vi "Write Experiment to TDMS Conversion Log.vi"(8 "error in (no error)":errorcluster, 10 "Additional Notes?":string, 11 "Conversion.lvclass":refnum<class "Conversion.lvclass">) -> (0 "error out":errorcluster, 2 "Log File Path":path, 3 "Conversion.lvclass out":refnum<class "Conversion.lvclass">)   [LabVIEW 2020, in "Conversion.lvclass"]
uses:
  Conversion.lvclass
  Conversion.lvclass/Conversion.ctl
  <userlib>/_OpenG.lib/array/array.llb/Remove Duplicates from 1D Array (Path)__ogtk.vi
  <userlib>/_OpenG.lib/file/file.llb/Strip Path - Arrays__ogtk.vi
panel:
  in  "OK":bool
  out "resulting string":string
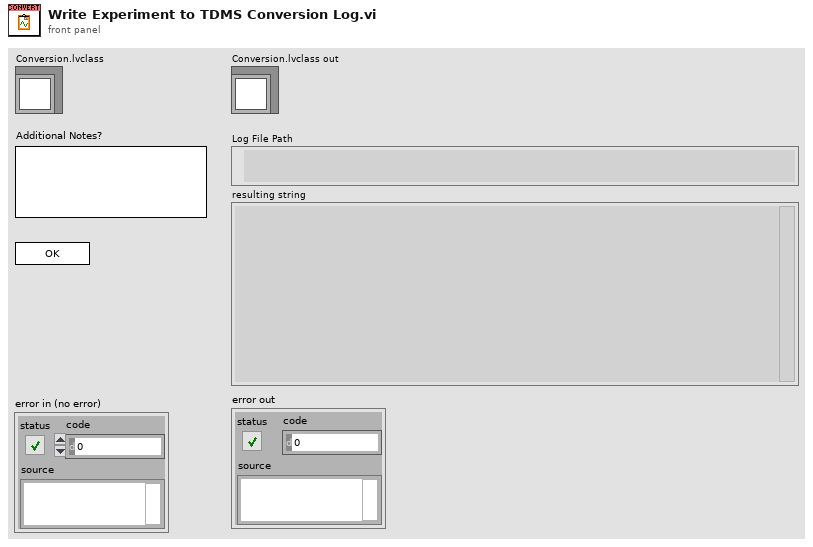
[diagram p1: front panel]
types:
  T1 = enum32{"Invalid", "Standard", "Closed", "Hidden", "Minimized", "Maximized"}
  T2 = enum32{"invalid app kind", "Development System", "Run Time System", "Student Edition", "Embedded LabVIEW", "Evaluation", "Custom"}
  T3 = cluster{"Core":cluster{"Current VI Reference":refnum<vi>, "Close Panel on Exit?":bool}, "Conversion.lvclass":refnum<class "Conversion.lvclass">, "Data.lvclass":refnum<class "Data.lvclass">, "Conversion Start time":timestamp, "Conversion End time":timestamp, "Archive End time":timestamp, "Original":path[], "Converted":path[], "Failed Conversions":path[], "Metadata":cluster{"Instrument":string, "Device":string, "Sample":string, "Experiment":string}, "Log":cluster{"Start Time":string, "Convert End Time":string, "Archive End Time":string, "string":string}}
  T4 = cluster{"Instrument":string, "Device":string, "Sample":string, "Experiment":string}
  T5 = cluster{"Start Time":string, "Convert End Time":string, "Archive End Time":string, "string":string}
  T6 = cluster{"Current VI Reference":refnum<vi>, "Close Panel on Exit?":bool}
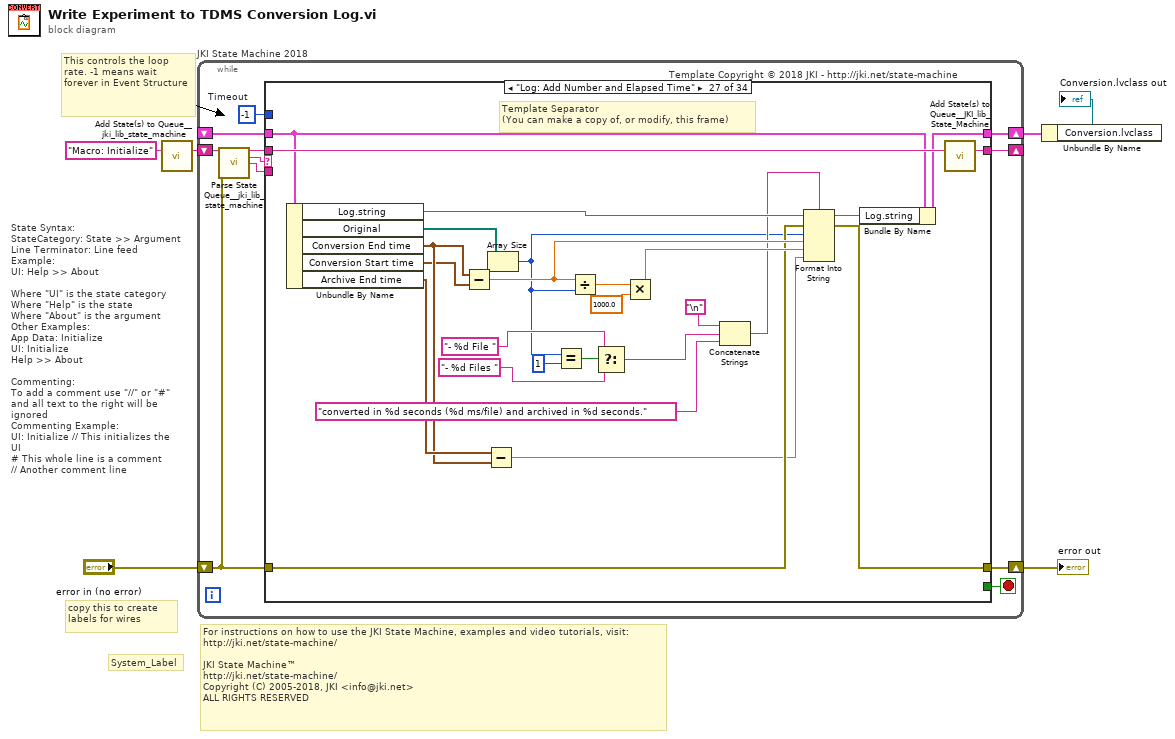
[diagram p0: block diagram]
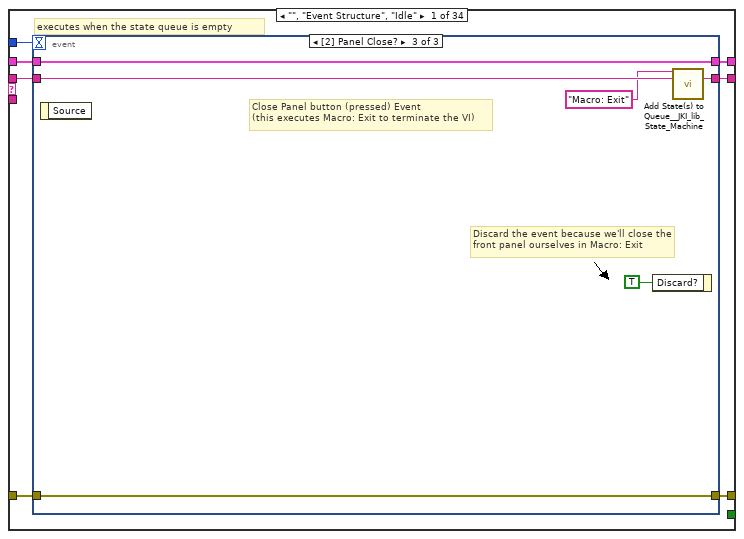
[diagram p2: hidden frame]
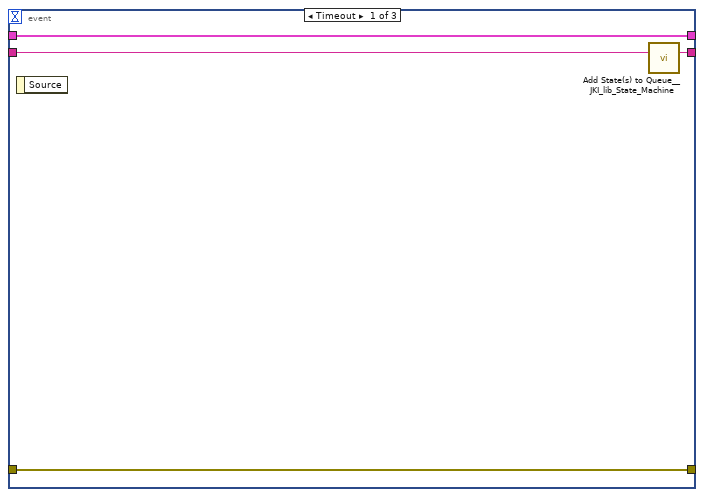
[diagram p3: hidden frame]
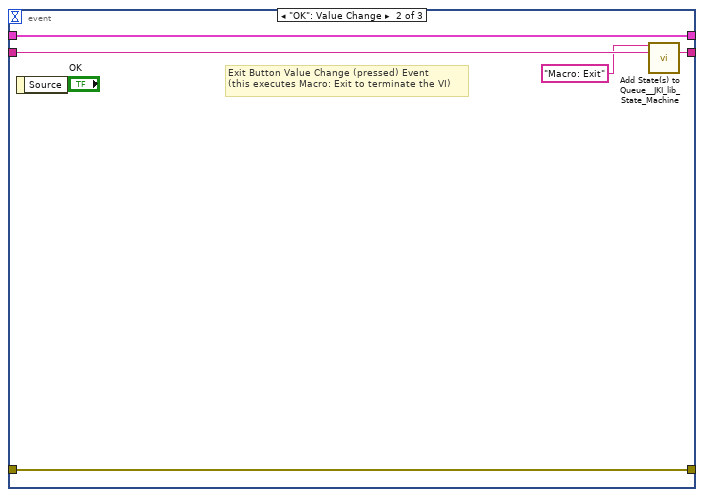
[diagram p4: hidden frame]
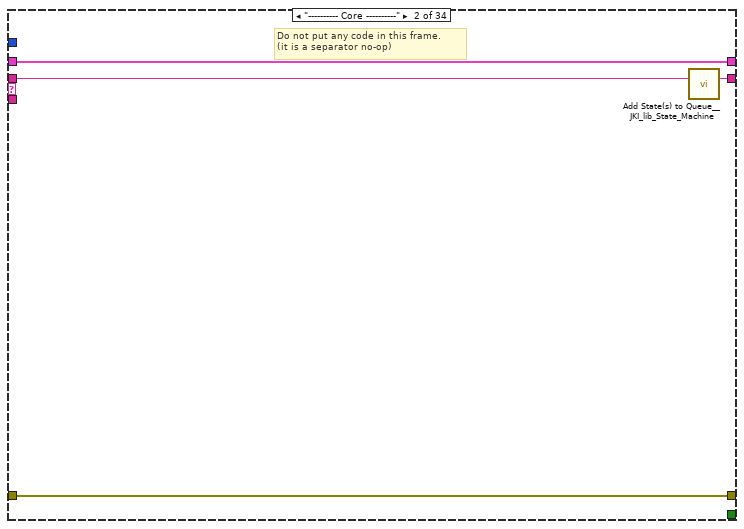
[diagram p5: hidden frame]
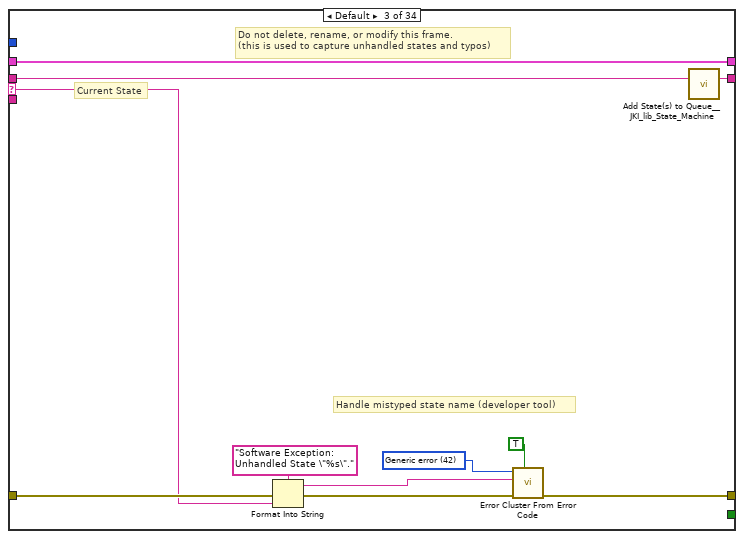
[diagram p6: hidden frame]
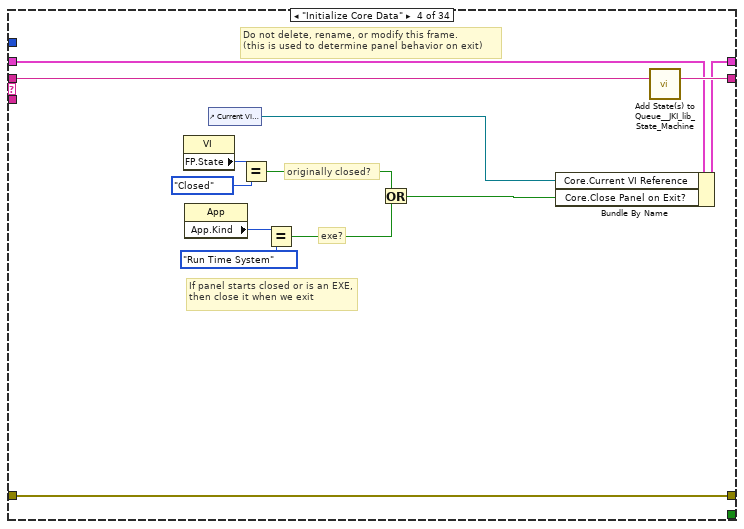
[diagram p7: hidden frame]
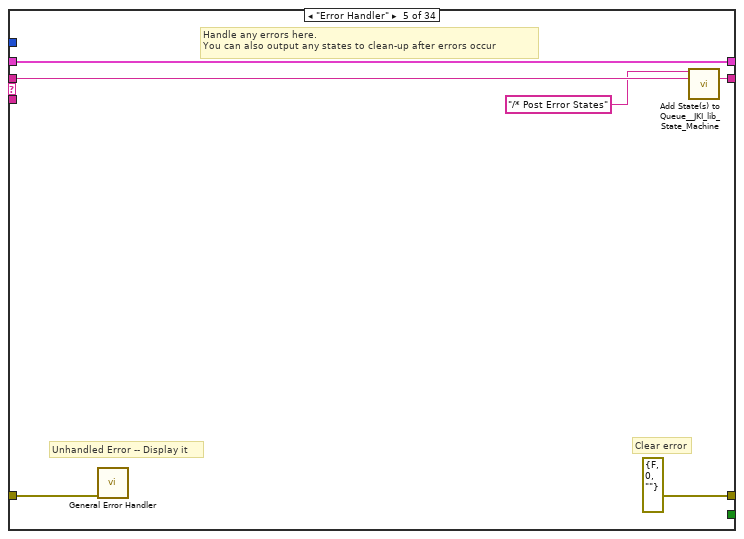
[diagram p8: hidden frame]
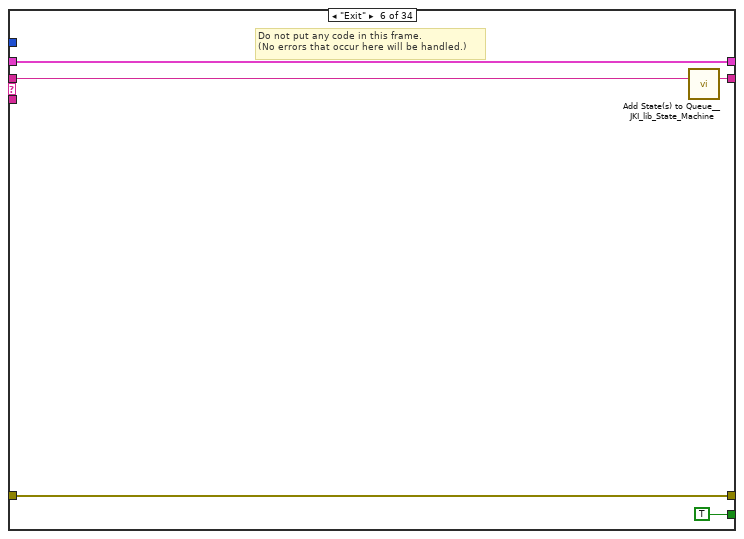
[diagram p9: hidden frame]
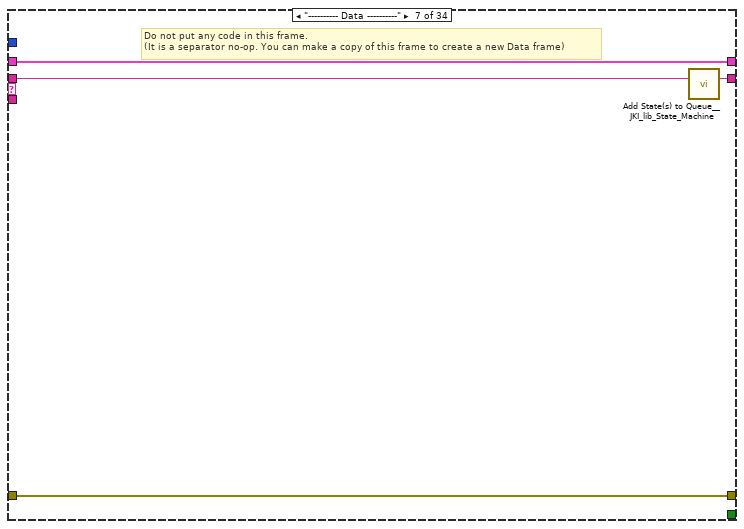
[diagram p10: hidden frame]
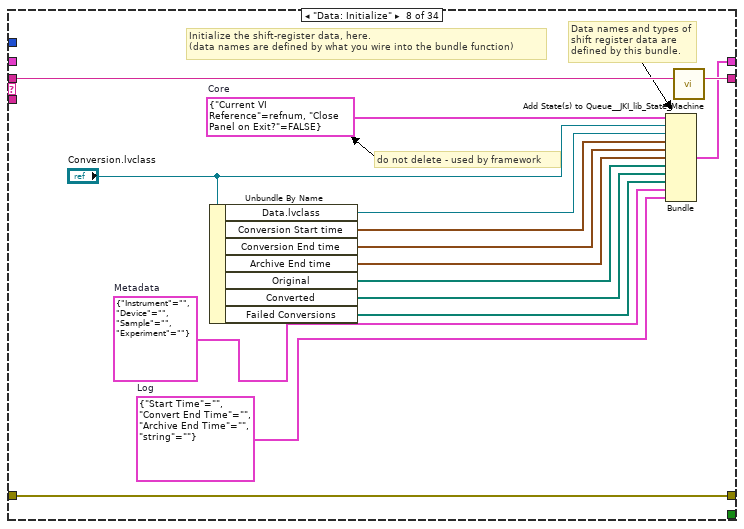
[diagram p11: hidden frame]
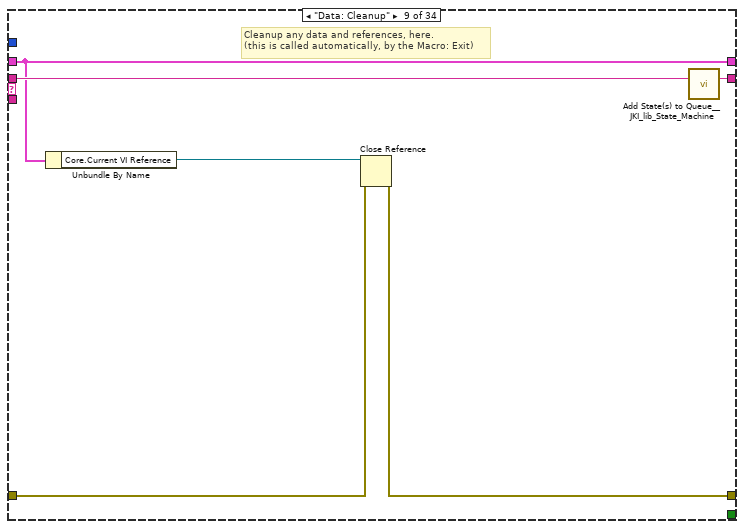
[diagram p12: hidden frame]
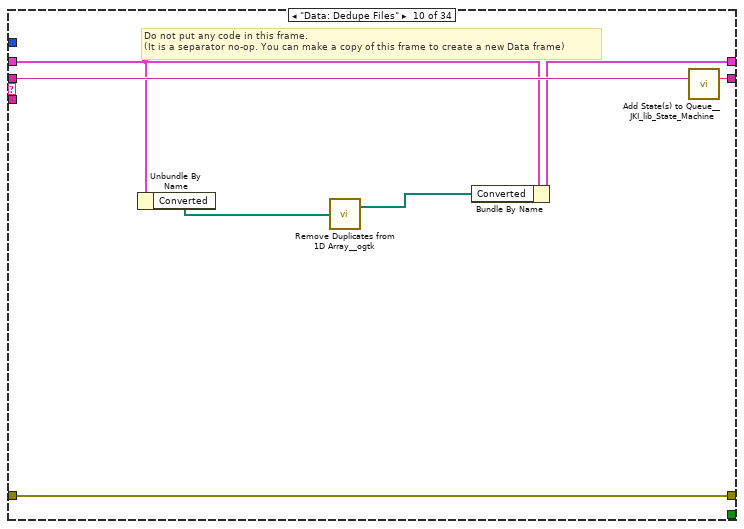
[diagram p13: hidden frame]
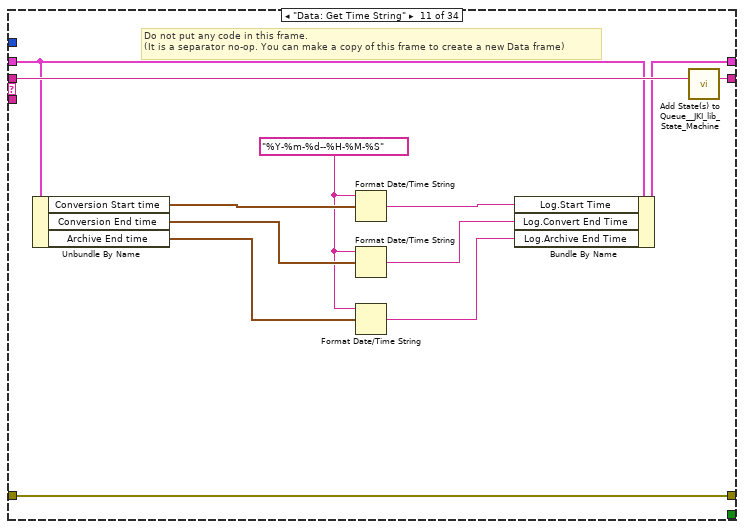
[diagram p14: hidden frame]
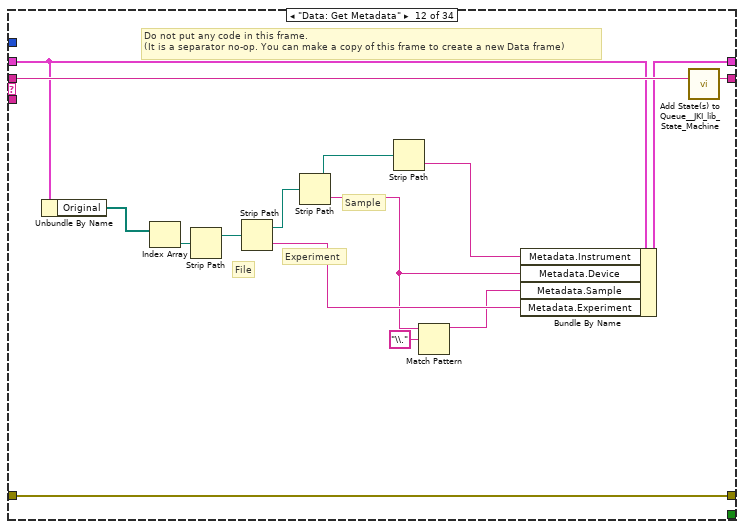
[diagram p15: hidden frame]
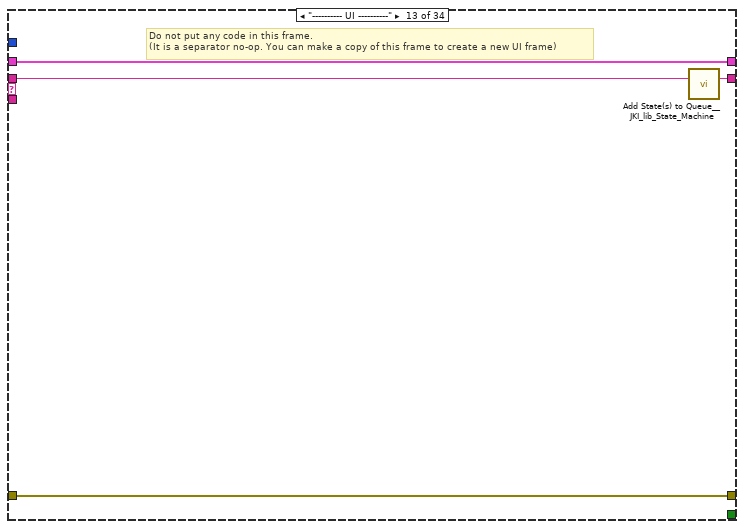
[diagram p16: hidden frame]
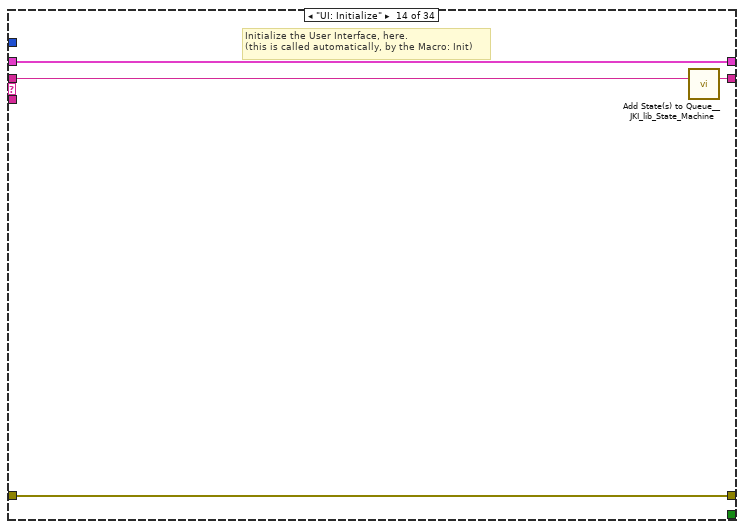
[diagram p17: hidden frame]
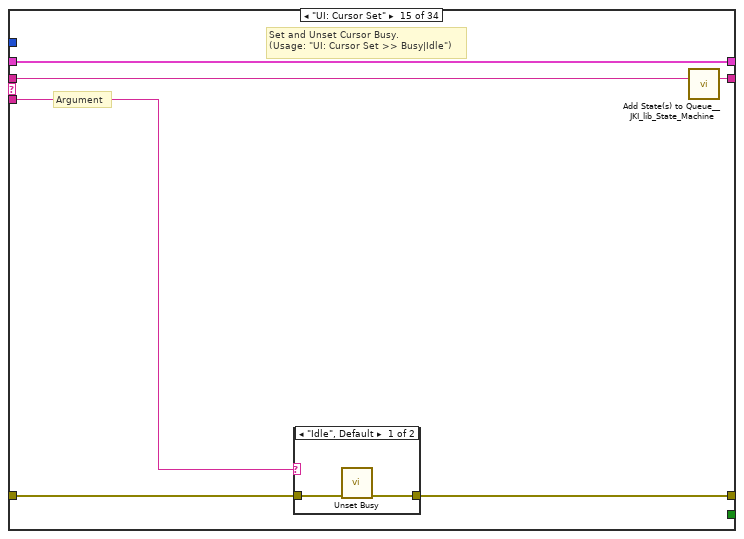
[diagram p18: hidden frame]
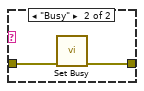
[diagram p19: hidden frame]
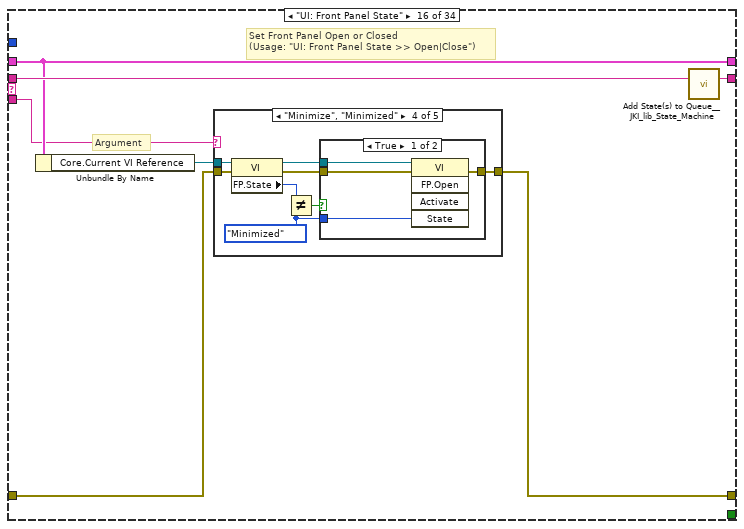
[diagram p20: hidden frame]
diagram:
  # "For instructions on how to use the JKI State Machine, examples and video tutorials, visit:\nhttp://jki.net/state-machine/\n\nJKI State Machine™\nhttp://jki.net/state-machine/\nCopyright (C) 2005-2018, JKI <info@jki.net>\nALL RIGHTS RESERVED"
  # "State Syntax:\nStateCategory: State >> Argument\nLine Terminator: Line feed\nExample:\nUI: Help >> About\n\nWhere \"UI\" is the state category\nWhere \"Help\" is the state\nWhere \"About\" is the argument\nOther Examples:\nApp Data: Initialize\nUI: Initialize\nHelp >> About\n\nCommenting:\nTo add a comment use \"//\" or \"#\" and all text to the right will be ignored\nCommenting Example:\nUI: Initialize // This initializes the UI\n# This whole line is a comment\n// Another comment line"
  # "copy this to create labels for wires"
  # "This controls the loop rate. -1 means wait forever in Event Structure"
  # "System_Label"
  n1 = call <vilib>:"Add State(s) to Queue__jki_lib_state_machine.vi"("State(s) in (\"\")"="Macro: Initialize") -> ("States Out"=w6:string)  [unwired: 14 in]
  n2 = while "JKI State Machine 2018" {
    shift-right: [w11] -> w2
    shift-left: _ -> [w10]
    shift-right: [w7] -> w4
    shift-left: "error in (no error)" -> [w8]
    shift-right: [w13] -> _
    shift-left: w6 -> [w14]
    stop <- w12 stop-if-true
    w9 = -1  # Timeout
    # "Template Copyright © 2018 JKI - http://jki.net/state-machine"
    n3 = call <vilib>:"Parse State Queue__jki_lib_state_machine.vi"("State Queue"=w14, "Error In (no error)"=w8) -> ("Remaining States"=w16:string, "Current State"=w17:string, "Arguments"=w15:string)  [unwired: 11 in]
    n4 = case shown="\"Log: Add Number and Elapsed Time\"" w17 {
      selector: w17 -> [_ _ w44 _ _ _ _ _ _ _ _ _ _ _ _ _ _ _ _ _ _ _ _ _ _ _ _ _ _ _ _ _ _ _]
      tunnel: w16 -> [w24 w43 w48 w67 w73 w78 w82 w97 w103 w110 w122 w137 w141 w145 w151 w162 w231 w236 w241 w251 w261 w265 w271 w281 w291 w301 w327 w339 w353 w388 w429 w447 w482 w508]
      tunnel: w15 -> [_ _ _ _ _ _ _ _ _ _ _ _ _ _ w146 w156 _ _ _ _ _ _ _ _ _ _ _ _ _ _ _ _ _ _]
      tunnel: w10 -> [w22 w40 w46 w60 w70 w76 w79 _ w98 w107 w119 w129 w138 w143 w149 w158 w228 w233 w238 w248 w259 w262 w268 w279 w289 w299 w325 w337 w351 w386 w427 w445 w480 w506]
      tunnel: w8 -> [w20 w41 w49 w64 w69 w75 w80 w94 w100 w108 w120 w135 w139 w142 w148 w160 w229 w234 w239 w249 w254 w263 w269 w273 w283 w293 w315 w332 w340 w381 w411 w441 w476 w497]
      tunnel: [w23 w42 w47 w66 w72 w77 w81 w96 w102 w109 w121 w136 w140 w144 w150 w161 w230 w235 w240 w250 w260 w264 w270 w280 w290 w300 w326 w338 w352 w387 w428 w446 w481 w507] -> w13
      tunnel: [_ _ _ _ _ TRUE _ _ _ _ _ _ _ _ _ _ _ _ _ _ _ _ _ _ _ _ _ _ _ _ _ _ _ _] -> w12
      tunnel: [w19 w40 w46 w65 w70 w76 w79 w95 w98 w105 w116 w128 w138 w143 w149 w158 w228 w233 w238 w248 w258 w262 w267 w278 w288 w298 w324 w336 w350 w385 w426 w444 w479 w506] -> w11
      tunnel: w9 -> [w18 _ _ _ _ _ _ _ _ _ _ _ _ _ _ _ _ _ _ _ _ _ _ _ _ _ _ _ _ _ _ _ _ _]
      tunnel: [w21 w41 w50 w64 errorcluster {"status"=FALSE, "code"=0, "source"=""} ("error out") w75 w80 w94 w99 w108 w120 w135 w139 w142 w147 w159 w229 w234 w239 w249 w253 w263 w269 w274 w282 w292 w316 w331 w346 w383 w422 w436 w475 w502] -> w7
      frame "", "Event Structure", "Idle" {
        # "executes when the state queue is empty"
        n5 = event shown="[2] Panel Close?" {
          selector: _ -> [_ _ _]
          dyn-events: _ -> [_ _ _]
          timeout: w18 -> [_ _ _]
          tunnel: w24 -> [w28 w33 w39]
          tunnel: [w27 w32 w38] -> w23
          tunnel: w22 -> [w25 w30 w36]
          tunnel: [w26 w31 w37] -> w21
          tunnel: w20 -> [w26 w31 w37]
          tunnel: [w25 w30 w36] -> w19
          event Timeout {
            n6 = event-data() -> ()  [unwired: 1 in, 1 out]
            n7 = call <vilib>:"Add State(s) to Queue__JKI_lib_State_Machine.vi"("State(s) in (\"\")"=w28) -> ("States Out"=w27:string)  [unwired: 14 in]
          }
          event "OK": Value Change {
            # "Exit Button Value Change (pressed) Event\n(this executes Macro: Exit to terminate the VI)"
            n8 = event-data() -> ()  [unwired: 1 in, 1 out]
            n9 = call <vilib>:"Add State(s) to Queue__JKI_lib_State_Machine.vi"("State(s) in Front (\"\")"="Macro: Exit", "State(s) in (\"\")"=w33) -> ("States Out"=w32:string)  [unwired: 13 in]
          }
          event Panel Close? {
            # "Discard the event because we'll close the front panel ourselves in Macro: Exit"
            # "Close Panel button (pressed) Event\n(this executes Macro: Exit to terminate the VI)"
            n10 = event-data() -> ()  [unwired: 1 in, 1 out]
            n11 = event-data("Discard?"=TRUE) -> ()  [unwired: 1 in, 1 out]
            n12 = call <vilib>:"Add State(s) to Queue__JKI_lib_State_Machine.vi"("State(s) in Front (\"\")"="Macro: Exit", "State(s) in (\"\")"=w39) -> ("States Out"=w38:string)  [unwired: 13 in]
          }
        }
      }
      frame "---------- Core ----------" {
        # "Do not put any code in this frame.\n(it is a separator no-op)"
        n13 = call <vilib>:"Add State(s) to Queue__JKI_lib_State_Machine.vi"("State(s) in (\"\")"=w43) -> ("States Out"=w42:string)  [unwired: 14 in]
      }
      frame Default {
        w53 = 42 items=["No error", "Argument error", "Memory is full", "Out of zone", "End of file", "File already open", "Generic file I/O error", "File not found", "File permission error", "Disk is full", "Duplicate path", "Too many files open", "System feature not enabled", "Resource file not found", "Cannot add resource", "Resource not found", "Image not found", "Image memory error", "Pen does not exist", "Config type invalid", "Config token not found", "Config parse error", "Config memory error", "Bad external code format", "Bad external code offset", "External code not present", "Null window", "Destroy window error", "Null menu", "Print aborted", "Bad print record", "Print driver error", "Windows error during printing", "Memory error during printing", "Print dialog error", "Generic print error", "Invalid device refnum", "Device not found", "Device parameter error", "Device unit error", "Cannot open device", "Device call aborted", "Generic error", "Cancelled by user", "Object ID too low", "Object ID too high", "Object not in heap", "Unknown heap", "Unknown object (invalid DefProc)", "Unknown object (DefProc not in table)", "Message out of range", "Invalid (null) method", "Unknown message", "Manager call not supported", "Bad address", "Network operation in progress", "Network operation timed out", "Connection is busy", "Network attribute not supported", "Network error", "Address in use", "System out of memory", "Connection aborted", "Connection refused", "Not connected", "Already connected", "Connection closed", "Initialization error (interapplication manager)", "Bad occurrence", "Wait on unbound occurrence handler", "Occurrence queue overflow", "Datalog type conflict", "Unused", "Unrecognized type (interapplication manager)", "Memory corrupt", "Failed to make temporary DLL", "Old CIN version", "Drag socket not found", "Failed to load drop-object", "Failed to register OLE object", "Failed to release OLE object", "Format specifier type mismatch", "Unknown format specifier", "Too few format specifiers", "Too many format specifiers", "Scan failed", "Newer CIN version", "Error converting to variant", "Runtime menu error", "Password tampered", "Variant attribute not found", "Incompatible variant data type", "Event data is not available", "Event Store is not present", "Occurrence is not found", "Event Queue is not created", "Event info is not available", "Refnum passed is NULL", "Error retrieving Class GUID", "Error retrieving CoClass GUID", "Error retrieving TypeLib GUID.", "Bad built application magic bytes.", "Specific driver is different from the specific driver associated with the Logical Name.", "There is no session opened to the class driver.", "Max Error", "MAX - Error with config objects", "MAX - Error loading configuration", "MAX - Group not supported"]
        # "Current State"
        # "Do not delete, rename, or modify this frame.\n(this is used to capture unhandled states and typos)"
        # "Handle mistyped state name (developer tool)"
        n14 = Format Into String(format string="Software Exception: Unhandled State \"%s\"." ("message"), error in=w49, w44) -> (resulting string=w52:string, error out=w51:errorcluster)  [unwired: 1 in]
        n15 = call <vilib>:"Error Cluster From Error Code.vi"("show call chain? (False)"=TRUE, "error in (no error)"=w51, "error message (\"\")"=w52, "error code (0)"=w53) -> ("error out"=w50:errorcluster)  [unwired: 5 in]
        n16 = call <vilib>:"Add State(s) to Queue__JKI_lib_State_Machine.vi"("State(s) in (\"\")"=w48) -> ("States Out"=w47:string)  [unwired: 14 in]
      }
      frame "Initialize Core Data" {
        # "Do not delete, rename, or modify this frame.\n(this is used to determine panel behavior on exit)"
        # "originally closed?"
        # "exe?"
        # "If panel starts closed or is an EXE, then close it when we exit"
        n17 = property class="VI"() -> ("FP.State"=w57:T1)  [unwired: 2 in, 2 out]
        n18 = property class="App"() -> ("App.Kind"=w63:T2)  [unwired: 2 in, 2 out]
        n19 = control-ref of="Current VI Reference"() -> (w58:refnum<vi>)
        n20 = Equal?(x=w57, y=T1."Closed" ("Front Panel Window:State")) -> (x = y?=w55:bool)
        n21 = Equal?(x=w63, y=T2."Run Time System" ("Application:Kind")) -> (x = y?=w61:bool)
        n22 = Or(x=w55, y=w61) -> (x .or. y?=w59:bool)
        n23 = Bundle By Name(cluster=w60, "Core.Current VI Reference"=w58, "Core.Close Panel on Exit?"=w59) -> (w65:T3)
        n24 = call <vilib>:"Add State(s) to Queue__JKI_lib_State_Machine.vi"("State(s) in (\"\")"=w67) -> ("States Out"=w66:string)  [unwired: 14 in]
      }
      frame "Error Handler" {
        # "Unhandled Error -- Display it"
        # "Handle any errors here.\nYou can also output any states to clean-up after errors occur"
        # "Clear error"
        n25 = call <vilib>:"General Error Handler.vi"("error in (no error)"=w69) -> ()  [unwired: 10 in, 5 out]
        n26 = call <vilib>:"Add State(s) to Queue__JKI_lib_State_Machine.vi"("State(s) in Front (\"\")"="/* Post Error States", "State(s) in (\"\")"=w73) -> ("States Out"=w72:string)  [unwired: 13 in]
      }
      frame "Exit" {
        # "Do not put any code in this frame.\n(No errors that occur here will be handled.)"
        n27 = call <vilib>:"Add State(s) to Queue__JKI_lib_State_Machine.vi"("State(s) in (\"\")"=w78) -> ("States Out"=w77:string)  [unwired: 14 in]
      }
      frame "---------- Data ----------" {
        # "Do not put any code in this frame.\n(It is a separator no-op. You can make a copy of this frame to create a new Data frame)"
        n28 = call <vilib>:"Add State(s) to Queue__JKI_lib_State_Machine.vi"("State(s) in (\"\")"=w82) -> ("States Out"=w81:string)  [unwired: 14 in]
      }
      frame "Data: Initialize" {
        w84 = T4 {"Instrument"="", "Device"="", "Sample"="", "Experiment"=""}  # Metadata
        w85 = T5 {"Start Time"="", "Convert End Time"="", "Archive End Time"="", "string"=""}  # Log
        w93 = T6 {"Current VI Reference"=refnum, "Close Panel on Exit?"=FALSE}  # Core
        # "do not delete - used by framework"
        # "Data names and types of shift register data are defined by this bundle."
        # "Initialize the shift-register data, here.\n(data names are defined by what you wire into the bundle function)"
        n29 = Unbundle By Name("Conversion.lvclass") -> ("Data.lvclass"=w92:refnum<class "Data.lvclass">, "Conversion Start time"=w91:timestamp, "Conversion End time"=w90:timestamp, "Archive End time"=w86:timestamp, "Original"=w88:path[], "Converted"=w87:path[], "Failed Conversions"=w89:path[])
        n30 = Bundle("Core"=w93, "Conversion.lvclass"="Conversion.lvclass", "Data.lvclass"=w92, "Conversion Start time"=w91, "Conversion End time"=w90, "Archive End time"=w86, "Original"=w88, "Converted"=w87, "Failed Conversions"=w89, "Metadata"=w84, "Log"=w85) -> (w95:T3)  [unwired: 1 in]
        n31 = call <vilib>:"Add State(s) to Queue__JKI_lib_State_Machine.vi"("State(s) in (\"\")"=w97) -> ("States Out"=w96:string)  [unwired: 14 in]
      }
      frame "Data: Cleanup" {
        # "Cleanup any data and references, here.\n(this is called automatically, by the Macro: Exit)"
        n32 = Unbundle By Name(w98) -> ("Core.Current VI Reference"=w101:refnum<vi>)
        n33 = Close Reference(reference=w101, error in (no error)=w100) -> (error out=w99:errorcluster)
        n34 = call <vilib>:"Add State(s) to Queue__JKI_lib_State_Machine.vi"("State(s) in (\"\")"=w103) -> ("States Out"=w102:string)  [unwired: 14 in]
      }
      frame "Data: Dedupe Files" {
        # "Do not put any code in this frame.\n(It is a separator no-op. You can make a copy of this frame to create a new Data frame)"
        n35 = Unbundle By Name(w107) -> ("Converted"=w106:path[])
        n36 = call-poly <userlib>:"Remove Duplicates from 1D Array__ogtk.vi"("Input Array"=w106) -> ("Output Array"=w104:path[])  [unwired: 1 out]
        n37 = Bundle By Name(cluster=w107, "Converted"=w104) -> (w105:T3)
        n38 = call <vilib>:"Add State(s) to Queue__JKI_lib_State_Machine.vi"("State(s) in (\"\")"=w110) -> ("States Out"=w109:string)  [unwired: 14 in]
      }
      frame "Data: Get Time String" {
        w112 = "%Y-%m-%d--%H-%M-%S" ("time format string (%c)")
        # "Do not put any code in this frame.\n(It is a separator no-op. You can make a copy of this frame to create a new Data frame)"
        n39 = Unbundle By Name(w119) -> ("Conversion Start time"=w118:timestamp, "Conversion End time"=w117:timestamp, "Archive End time"=w113:timestamp)
        n40 = Format Date/Time String(time format string (%c)=w112, seconds (now)=w118) -> (date/time string=w115:string)  [unwired: 1 in]
        n41 = Format Date/Time String(time format string (%c)=w112, seconds (now)=w117) -> (date/time string=w114:string)  [unwired: 1 in]
        n42 = Format Date/Time String(time format string (%c)=w112, seconds (now)=w113) -> (date/time string=w111:string)  [unwired: 1 in]
        n43 = Bundle By Name(cluster=w119, "Log.Start Time"=w115, "Log.Convert End Time"=w114, "Log.Archive End Time"=w111) -> (w116:T3)
        n44 = call <vilib>:"Add State(s) to Queue__JKI_lib_State_Machine.vi"("State(s) in (\"\")"=w122) -> ("States Out"=w121:string)  [unwired: 14 in]
      }
      frame "Data: Get Metadata" {
        # "Sample"
        # "Experiment"
        # "File"
        # "Do not put any code in this frame.\n(It is a separator no-op. You can make a copy of this frame to create a new Data frame)"
        n45 = Unbundle By Name(w129) -> ("Original"=w130:path[])
        n46 = Index Array(array=w130) -> (element=w133:path)  [unwired: 1 in]
        n47 = Strip Path(path=w133) -> (stripped path=w132:path)  [unwired: 1 out]
        n48 = Strip Path(path=w132) -> (stripped path=w134:path, name=w126:string)
        n49 = Strip Path(path=w134) -> (stripped path=w131:path, name=w125:string)
        n50 = Strip Path(path=w131) -> (name=w127:string)  [unwired: 1 out]
        n51 = Match Pattern(string=w125, regular expression="\\.") -> (before substring=w123:string)  [unwired: 1 in, 3 out]
        n52 = Bundle By Name(cluster=w129, "Metadata.Instrument"=w127, "Metadata.Device"=w125, "Metadata.Sample"=w123, "Metadata.Experiment"=w126) -> (w128:T3)
        n53 = call <vilib>:"Add State(s) to Queue__JKI_lib_State_Machine.vi"("State(s) in (\"\")"=w137) -> ("States Out"=w136:string)  [unwired: 14 in]
      }
      frame "---------- UI ----------" {
        # "Do not put any code in this frame.\n(It is a separator no-op. You can make a copy of this frame to create a new UI frame)"
        n54 = call <vilib>:"Add State(s) to Queue__JKI_lib_State_Machine.vi"("State(s) in (\"\")"=w141) -> ("States Out"=w140:string)  [unwired: 14 in]
      }
      frame "UI: Initialize" {
        # "Initialize the User Interface, here.\n(this is called automatically, by the Macro: Init)"
        n55 = call <vilib>:"Add State(s) to Queue__JKI_lib_State_Machine.vi"("State(s) in (\"\")"=w145) -> ("States Out"=w144:string)  [unwired: 14 in]
      }
      frame "UI: Cursor Set" {
        # "Argument"
        # "Set and Unset Cursor Busy.\n(Usage: \"UI: Cursor Set >> Busy|Idle\")"
        n56 = case shown="\"Idle\", Default" w146 {
          tunnel: w148 -> [w153 w155]
          tunnel: [w152 w154] -> w147
          frame "Idle", Default {
            n57 = call <vilib>:"Unset Busy.vi"("error in (no error)"=w153) -> ("error out"=w152:errorcluster)  [unwired: 10 in]
          }
          frame "Busy" {
            n58 = call <vilib>:"Set Busy.vi"("error in (no error)"=w155) -> ("error out"=w154:errorcluster)  [unwired: 9 in, 1 out]
          }
        }
        n59 = call <vilib>:"Add State(s) to Queue__JKI_lib_State_Machine.vi"("State(s) in (\"\")"=w151) -> ("States Out"=w150:string)  [unwired: 14 in]
      }
      frame "UI: Front Panel State" {
        # "Argument"
        # "Set Front Panel Open or Closed\n(Usage: \"UI: Front Panel State >> Open|Close\")"
        n60 = Unbundle By Name(w158) -> ("Core.Current VI Reference"=w157:refnum<vi>)
        n61 = case shown="\"Minimize\", \"Minimized\"" w156 {
          tunnel: w160 -> [w168 w183 w194 w207 w220]
          tunnel: [w170 w184 w196 w209 w222] -> w159
          tunnel: w157 -> [w169 w181 w195 w208 w221]
          frame "Open", "Standard", Default {
            w163 = T1."Standard" ("State")
            n62 = property class="VI"(reference=w169, error in=w168) -> (reference out=w166:refnum<vi>, error out=w167:errorcluster, "FP.State"=w165:T1)
            n63 = Not Equal?(x=w165, y=w163) -> (x != y?=w164:bool)
            n64 = case shown="True" w164 {
              tunnel: [w174 w176] -> w170
              tunnel: w167 -> [w173 w176]
              tunnel: w166 -> [w172 _]
              tunnel: w163 -> [w171 _]
              frame True {
                n65 = invoke class="VI" method="FP.Open"(reference=w172, error in=w173, "Activate"=TRUE, "State"=w171) -> (error out=w174:errorcluster)  [unwired: 1 in, 4 out]
              }
              frame False {
              }
            }
          }
          frame "Close", "Closed" {
            n66 = property class="VI"(reference=w181, error in=w183) -> (reference out=w180:refnum<vi>, error out=w182:errorcluster, "FP.State"=w178:T1)
            n67 = Not Equal?(x=w178, y=T1."Closed" ("Front Panel Window:State")) -> (x != y?=w177:bool)
            n68 = case shown="True" w177 {
              tunnel: [w185 w188] -> w184
              tunnel: w182 -> [w185 w187]
              tunnel: w180 -> [_ w186]
              frame False {
              }
              frame True {
                n69 = invoke class="VI" method="FP.Close"(reference=w186, error in=w187) -> (error out=w188:errorcluster)  [unwired: 1 in, 2 out]
              }
            }
          }
          frame "Hidden", "Hide" {
            w189 = T1."Hidden" ("State")
            n70 = property class="VI"(reference=w195, error in=w194) -> (reference out=w192:refnum<vi>, error out=w193:errorcluster, "FP.State"=w191:T1)
            n71 = Not Equal?(x=w191, y=w189) -> (x != y?=w190:bool)
            n72 = case shown="True" w190 {
              tunnel: [w200 w201] -> w196
              tunnel: w193 -> [w199 w201]
              tunnel: w192 -> [w198 _]
              tunnel: w189 -> [w197 _]
              frame True {
                n73 = invoke class="VI" method="FP.Open"(reference=w198, error in=w199, "State"=w197) -> (error out=w200:errorcluster)  [unwired: 2 in, 4 out]
              }
              frame False {
              }
            }
          }
          frame "Minimize", "Minimized" {
            w202 = T1."Minimized" ("State")
            n74 = property class="VI"(reference=w208, error in=w207) -> (reference out=w205:refnum<vi>, error out=w206:errorcluster, "FP.State"=w204:T1)
            n75 = Not Equal?(x=w204, y=w202) -> (x != y?=w203:bool)
            n76 = case shown="True" w203 {
              tunnel: [w213 w214] -> w209
              tunnel: w206 -> [w212 w214]
              tunnel: w205 -> [w211 _]
              tunnel: w202 -> [w210 _]
              frame True {
                n77 = invoke class="VI" method="FP.Open"(reference=w211, error in=w212, "State"=w210) -> (error out=w213:errorcluster)  [unwired: 2 in, 4 out]
              }
              frame False {
              }
            }
          }
          frame "Maximize", "Maximized" {
            w215 = T1."Maximized" ("State")
            n78 = property class="VI"(reference=w221, error in=w220) -> (reference out=w218:refnum<vi>, error out=w219:errorcluster, "FP.State"=w217:T1)
            n79 = Not Equal?(x=w217, y=w215) -> (x != y?=w216:bool)
            n80 = case shown="True" w216 {
              tunnel: [w226 w227] -> w222
              tunnel: w219 -> [w225 w227]
              tunnel: w218 -> [w224 _]
              tunnel: w215 -> [w223 _]
              frame True {
                n81 = invoke class="VI" method="FP.Open"(reference=w224, error in=w225, "State"=w223) -> (error out=w226:errorcluster)  [unwired: 2 in, 4 out]
              }
              frame False {
              }
            }
          }
        }
        n82 = call <vilib>:"Add State(s) to Queue__JKI_lib_State_Machine.vi"("State(s) in (\"\")"=w162) -> ("States Out"=w161:string)  [unwired: 14 in]
      }
      frame "---------- Macro ----------" {
        # "Do not put any code in this frame.\n(It is a separator no-op. You can make a copy of this frame to create a new Macro frame)"
        n83 = call <vilib>:"Add State(s) to Queue__JKI_lib_State_Machine.vi"("State(s) in (\"\")"=w231) -> ("States Out"=w230:string)  [unwired: 14 in]
      }
      frame "Macro: Initialize" {
        w232 = "Data: Initialize\nInitialize Core Data\nUI: Initialize\nUI: Front Panel State >> Open\nMacro: Log\nMacro: Exit"  # Data: Initialize Initialize Core Data UI: Initialize UI: Front Panel State >> Open Macro: Log Macro: Exit
        # "Initialization Macro\n(This is called once, when the VI starts)"
        n84 = call <vilib>:"Add State(s) to Queue__JKI_lib_State_Machine.vi"("State(s) in Front (\"\")"=w232, "State(s) in (\"\")"=w236) -> ("States Out"=w235:string)  [unwired: 13 in]
      }
      frame "Macro: Log" {
        # "Initialization Macro\n(This is called once, when the VI starts)"
        n85 = call <vilib>:"Add State(s) to Queue__JKI_lib_State_Machine.vi"("State(s) in Front (\"\")"="Log: Temp\nData: Dedupe Files\nData: Get Time String\nData: Get Metadata\nLog: Initialize\nLog: Add Start Time\nLog: Add Convert End Time\nLog: Add Archive End Time\nLog: Add Number and Elapsed Time\nLog: Add Original Folder Name\nLog: Add Converted Folder Name\nLog: Add Number of Files\nLog: Add File Sizes\nLog: Add Notes\nLog: Add Files\nLog: Write File", "State(s) in (\"\")"=w241) -> ("States Out"=w240:string)  [unwired: 13 in]
      }
      frame "Macro: Exit" {
        # "Exit Macro\n(This is called once, when the VI exits)"
        n86 = Unbundle By Name(w248) -> ("Core.Close Panel on Exit?"=w247:bool)
        n87 = Select(t="UI: Front Panel State >> Close", s=w247, f="") -> (s? t:f=w244:string)
        n88 = call <vilib>:"Add State(s) to Queue__JKI_lib_State_Machine.vi"("State(s) in (\"\")"=w244, "State(s) at Back (\"\")"="Data: Cleanup\nExit") -> ("States Out"=w242:string)  [unwired: 13 in]
        n89 = call <vilib>:"Add State(s) to Queue__JKI_lib_State_Machine.vi"("State(s) in Front (\"\")"=w242, "State(s) in (\"\")"=w251) -> ("States Out"=w250:string)  [unwired: 13 in]
      }
      frame "---------- Log ----------" {
        # "Template Separator\n(You can make a copy of, or modify, this frame)"
        n90 = Unbundle By Name(w259) -> ("Log.string"=w256:string)
        n91 = Format Into String(format string="\n%s", initial string=w256, error in=w254, "" ("input 1")) -> (resulting string=w255:string, error out=w253:errorcluster)
        n92 = Bundle By Name(cluster=w259, "Log.string"=w255) -> (w258:T3)
        n93 = call <vilib>:"Add State(s) to Queue__JKI_lib_State_Machine.vi"("State(s) in (\"\")"=w261) -> ("States Out"=w260:string)  [unwired: 14 in]
      }
      frame "Log: Temp" {
        # "Your code here.\n(You can make a copy of, or modify, this frame)"
        n94 = call <vilib>:"Add State(s) to Queue__JKI_lib_State_Machine.vi"("State(s) in (\"\")"=w265) -> ("States Out"=w264:string)  [unwired: 14 in]
      }
      frame "Log: Initialize" {
        w266 = "Data File Conversion Summary"  # new
        # "Template Separator\n(You can make a copy of, or modify, this frame)"
        n95 = Bundle By Name(cluster=w268, "Log.string"=w266) -> (w267:T3)
        n96 = call <vilib>:"Add State(s) to Queue__JKI_lib_State_Machine.vi"("State(s) in (\"\")"=w271) -> ("States Out"=w270:string)  [unwired: 14 in]
      }
      frame "Log: Add Start Time" {
        # "Template Separator\n(You can make a copy of, or modify, this frame)"
        n97 = Unbundle By Name(w279) -> ("Log.string"=w276:string, "Log.Start Time"=w272:string)
        n98 = Format Into String(format string="\n- Start Time: %s", initial string=w276, error in=w273, w272) -> (resulting string=w275:string, error out=w274:errorcluster)
        n99 = Bundle By Name(cluster=w279, "Log.string"=w275) -> (w278:T3)
        n100 = call <vilib>:"Add State(s) to Queue__JKI_lib_State_Machine.vi"("State(s) in (\"\")"=w281) -> ("States Out"=w280:string)  [unwired: 14 in]
      }
      frame "Log: Add Convert End Time" {
        # "Template Separator\n(You can make a copy of, or modify, this frame)"
        n101 = Unbundle By Name(w289) -> ("Log.string"=w286:string, "Log.Convert End Time"=w285:string)
        n102 = Format Into String(format string="\n- End Time: %s", initial string=w286, error in=w283, w285) -> (resulting string=w284:string, error out=w282:errorcluster)
        n103 = Bundle By Name(cluster=w289, "Log.string"=w284) -> (w288:T3)
        n104 = call <vilib>:"Add State(s) to Queue__JKI_lib_State_Machine.vi"("State(s) in (\"\")"=w291) -> ("States Out"=w290:string)  [unwired: 14 in]
      }
      frame "Log: Add Archive End Time" {
        # "Template Separator\n(You can make a copy of, or modify, this frame)"
        n105 = Unbundle By Name(w299) -> ("Log.string"=w296:string, "Log.Archive End Time"=w295:string)
        n106 = Format Into String(format string="\n- Archive End Time: %s", initial string=w296, error in=w293, w295) -> (resulting string=w294:string, error out=w292:errorcluster)
        n107 = Bundle By Name(cluster=w299, "Log.string"=w294) -> (w298:T3)
        n108 = call <vilib>:"Add State(s) to Queue__JKI_lib_State_Machine.vi"("State(s) in (\"\")"=w301) -> ("States Out"=w300:string)  [unwired: 14 in]
      }
      frame "Log: Add Number and Elapsed Time" {
        # "Template Separator\n(You can make a copy of, or modify, this frame)"
        n109 = Unbundle By Name(w325) -> ("Log.string"=w323:string, "Original"=w322:path[], "Conversion End time"=w304:timestamp, "Conversion Start time"=w303:timestamp, "Archive End time"=w305:timestamp)
        n110 = Subtract(x=w304, y=w303) -> (x-y=w319:dbl)
        n111 = Subtract(x=w305, y=w304) -> (x-y=w302:dbl)
        n112 = Array Size(array=w322) -> (size(s)=w306:i32)
        n113 = Equal?(x=w306, y=1) -> (x = y?=w313:bool)
        n114 = Divide(x=w319, y=w306) -> (x/y=w320:dbl)
        n115 = Select(t="- %d File " ("format string"), s=w313, f="- %d Files " ("format string")) -> (s? t:f=w308:string)
        n116 = Multiply(x=w320, y=1000.0) -> (x*y=w317:dbl)
        n117 = Concatenate Strings("\n", w308, "converted in %d seconds (%d ms/file) and archived in %d seconds." ("format string")) -> (w307:string)
        n118 = Format Into String(format string=w307, initial string=w323, error in=w315, w306, w319, w317, w302) -> (resulting string=w318:string, error out=w316:errorcluster)
        n119 = Bundle By Name(cluster=w325, "Log.string"=w318) -> (w324:T3)
        n120 = call <vilib>:"Add State(s) to Queue__JKI_lib_State_Machine.vi"("State(s) in (\"\")"=w327) -> ("States Out"=w326:string)  [unwired: 14 in]
      }
      frame "Log: Add Original Folder Name" {
        # "Template Separator\n(You can make a copy of, or modify, this frame)"
        n121 = Unbundle By Name(w337) -> ("Log.string"=w334:string, "Original"=w329:path[])
        n122 = Index Array(array=w329) -> (element=w330:path)  [unwired: 1 in]
        n123 = Strip Path(path=w330) -> (stripped path=w328:path)  [unwired: 1 out]
        n124 = Format Into String(format string="\n- Original Folder: %s", initial string=w334, error in=w332, w328) -> (resulting string=w333:string, error out=w331:errorcluster)
        n125 = Bundle By Name(cluster=w337, "Log.string"=w333) -> (w336:T3)
        n126 = call <vilib>:"Add State(s) to Queue__JKI_lib_State_Machine.vi"("State(s) in (\"\")"=w339) -> ("States Out"=w338:string)  [unwired: 14 in]
      }
      frame "Log: Add Converted Folder Name" {
        # "Template Separator\n(You can make a copy of, or modify, this frame)"
        n127 = Unbundle By Name(w351) -> ("Log.string"=w341:string, "Converted"=w347:path[])
        n128 = Path To String(path=w347) -> (string=w343:string[])
        n129 = for {
          tunnel: w343 -> [w355] mode=indexing
          tunnel: [w354] -> w345 mode=indexing
          n130 = Concatenate Strings("  - " ("format string"), w355) -> (w354:string)
        }
        n131 = call <userlib>:"1D Array to String__ogtk.vi"("delimiter (Tab)"="\n", "Array of Strings"=w345) -> ("delimited string"=w342:string)  [unwired: 9 in]
        n132 = Format Into String(format string="\n- Converted File(s):\n%s", initial string=w341, error in=w340, w342) -> (resulting string=w348:string, error out=w346:errorcluster)
        n133 = Bundle By Name(cluster=w351, "Log.string"=w348) -> (w350:T3)
        n134 = call <vilib>:"Add State(s) to Queue__JKI_lib_State_Machine.vi"("State(s) in (\"\")"=w353) -> ("States Out"=w352:string)  [unwired: 14 in]
      }
      frame "Log: Add Number of Files" {
        # "Template Separator\n(You can make a copy of, or modify, this frame)"
        n135 = Unbundle By Name(w386) -> ("Log.string"=w384:string, "Original"=w382:path[], "Converted"=w367:path[])
        n136 = Array Size(array=w382) -> (size(s)=w377:i32)
        n137 = Array Size(array=w367) -> ()  [unwired: 1 out]
        n138 = for {
          tunnel: w367 -> [w394] mode=indexing
          tunnel: [w390] -> w366 mode=indexing if=w390
          tunnel: [w389] -> w365 mode=indexing if=w389
          n139 = call <vilib>:"Get File Extension.vi"("file"=w394) -> ("unmodified file extension"=w391:string)  [unwired: 6 in, 4 out]
          n140 = Equal?(x=w391, y="tdms") -> (x = y?=w390:bool)
          n141 = Equal?(x=w391, y="zip") -> (x = y?=w389:bool)
        }
        n142 = Equal?(x=w377, y=1) -> (x = y?=w375:bool)
        n143 = Select(t="- %d ITX file " ("format string"), s=w375, f="- %d ITX files " ("format string")) -> (s? t:f=w374:string)
        n144 = Array Size(array=w366) -> (size(s)=w358:i32)
        n145 = Array Size(array=w365) -> (size(s)=w357:i32)
        n146 = Equal?(x=w357, y=1) -> (x = y?=w362:bool)
        n147 = Equal?(x=w358, y=1) -> (x = y?=w371:bool)
        n148 = Select(t="and %d ZIP file" ("format string"), s=w362, f="and %d ZIP files" ("format string")) -> (s? t:f=w360:string)
        n149 = Select(t="converted to %d TDMS file " ("format string"), s=w371, f="converted to %d TDMS files " ("format string")) -> (s? t:f=w361:string)
        n150 = Concatenate Strings("\n", w374, w361, w360) -> (w378:string)
        n151 = Format Into String(format string=w378, initial string=w384, error in=w381, w377, w358, w357) -> (resulting string=w380:string, error out=w383:errorcluster)
        n152 = Bundle By Name(cluster=w386, "Log.string"=w380) -> (w385:T3)
        n153 = call <vilib>:"Add State(s) to Queue__JKI_lib_State_Machine.vi"("State(s) in (\"\")"=w388) -> ("States Out"=w387:string)  [unwired: 14 in]
      }
      frame "Log: Add File Sizes" {
        w395 = "MB"
        w396 = "KB"
        w403 = i64 1048576 ("y")
        w406 = i64 1048576 ("y")
        # "Template Separator\n(You can make a copy of, or modify, this frame)"
        n154 = Unbundle By Name(w427) -> ("Log.string"=w424:string, "Original"=w420:path[], "Converted"=w417:path[])
        n155 = for {
          tunnel: [w433] -> w421 mode=indexing
          tunnel: w420 -> [w432] mode=indexing
          n156 = File/Directory Info(path=w432) -> (size=w433:i64)  [unwired: 1 in, 6 out]
        }
        n157 = for {
          tunnel: [w431] -> w418 mode=indexing
          tunnel: w417 -> [w430] mode=indexing
          n158 = File/Directory Info(path=w430) -> (size=w431:i64)  [unwired: 1 in, 6 out]
        }
        n159 = Add Array Elements(numeric array=w421) -> (sum=w410:i64)
        n160 = Add Array Elements(numeric array=w418) -> (sum=w407:i64)
        n161 = Less Or Equal?(x=w407, y=w403) -> (x <= y?=w399:bool)
        n162 = Less Or Equal?(x=w410, y=w406) -> (x <= y?=w400:bool)
        n163 = Select(t=i64 1024, s=w400, f=w406) -> (s? t:f=w408:i64)
        n164 = Select(t=i64 1024, s=w399, f=w403) -> (s? t:f=w405:i64)
        n165 = Select(t=w396, s=w400, f=w395) -> (s? t:f=w398:string)
        n166 = Select(t=w396, s=w399, f=w395) -> (s? t:f=w397:string)
        n167 = Divide(x=w410, y=w408) -> (x/y=w412:dbl)
        n168 = Divide(x=w407, y=w405) -> (x/y=w413:dbl)
        n169 = To Long Integer(number=w412) -> (32bit integer=w419:i32)
        n170 = To Long Integer(number=w413) -> (32bit integer=w401:i32)
        n171 = Divide(x=w413, y=w412) -> (x/y=w414:dbl)
        n172 = Multiply(x=w414, y=100.0) -> (x*y=w416:dbl)
        n173 = To Long Integer(number=w416) -> (32bit integer=w402:i32)
        n174 = Format Into String(format string="\n- Original Folder Size: %d %s\n- Converted Folder Size: %d %s\n- The Converted File is %d\\% of the size of the Original", initial string=w424, error in=w411, w419, w398, w401, w397, w402) -> (resulting string=w423:string, error out=w422:errorcluster)
        n175 = Bundle By Name(cluster=w427, "Log.string"=w423) -> (w426:T3)
        n176 = call <vilib>:"Add State(s) to Queue__JKI_lib_State_Machine.vi"("State(s) in (\"\")"=w429) -> ("States Out"=w428:string)  [unwired: 14 in]
      }
      frame "Log: Add Notes" {
        # "Template Separator\n(You can make a copy of, or modify, this frame)"
        n177 = call <userlib>:"Multi-line String to Array__ogtk.vi"("string"="Additional Notes?") -> ("lines"=w440:string[])
        n178 = Empty String/Path?(string/path="Additional Notes?") -> (empty?=w434:bool)
        n179 = Unbundle By Name(w445) -> ("Log.string"=w443:string)
        n180 = for {
          tunnel: w440 -> [w457] mode=indexing
          tunnel: [w456] -> w439 mode=indexing
          n181 = Concatenate Strings("  - " ("format string"), w457) -> (w456:string)
        }
        n182 = call <userlib>:"1D Array to String__ogtk.vi"("delimiter (Tab)"="\n", "Array of Strings"=w439) -> ("delimited string"=w437:string)  [unwired: 9 in]
        n183 = case shown="True" w434 {
          tunnel: w443 -> [w452 w455]
          tunnel: [w451 w455] -> w442
          tunnel: w441 -> [w450 w454]
          tunnel: w437 -> [w449 _]
          tunnel: [w448 w454] -> w436
          frame False {
            n184 = Format Into String(format string="\n- Notes:\n%s", initial string=w452, error in=w450, w449) -> (resulting string=w451:string, error out=w448:errorcluster)
          }
          frame True {
          }
        }
        n185 = Bundle By Name(cluster=w445, "Log.string"=w442) -> (w444:T3)
        n186 = call <vilib>:"Add State(s) to Queue__JKI_lib_State_Machine.vi"("State(s) in (\"\")"=w447) -> ("States Out"=w446:string)  [unwired: 14 in]
      }
      frame "Log: Add Files" {
        # "Template Separator\n(You can make a copy of, or modify, this frame)"
        n187 = Unbundle By Name(w480) -> ("Log.string"=w477:string, "Converted"=w473:path[], "Failed Conversions"=w472:path[], "Original"=w471:path[])
        n188 = call-poly <userlib>:"Strip Path__ogtk.vi"("path"=w471) -> ("name"=w468:string[])  [unwired: 1 out]
        n189 = call-poly <userlib>:"Strip Path__ogtk.vi"("path"=w472) -> ("name"=w462:string[])  [unwired: 1 out]
        n190 = call-poly <userlib>:"Strip Path__ogtk.vi"("path"=w473) -> ("name"=w463:string[])  [unwired: 1 out]
        n191 = for {
          tunnel: w463 -> [w484] mode=indexing
          tunnel: [w483] -> w465 mode=indexing
          n192 = Concatenate Strings("  - " ("format string"), w484) -> (w483:string)
        }
        n193 = for {
          tunnel: w462 -> [w487] mode=indexing
          tunnel: [w486] -> w466 mode=indexing
          n194 = Concatenate Strings("  - " ("format string"), w487) -> (w486:string)
        }
        n195 = for {
          tunnel: w468 -> [w490] mode=indexing
          tunnel: [w489] -> w470 mode=indexing
          n196 = Concatenate Strings("  - " ("format string"), w490) -> (w489:string)
        }
        n197 = call <userlib>:"1D Array to String__ogtk.vi"("delimiter (Tab)"="\n", "Array of Strings"=w465) -> ("delimited string"=w461:string)  [unwired: 9 in]
        n198 = call <userlib>:"1D Array to String__ogtk.vi"("delimiter (Tab)"="\n", "Array of Strings"=w466) -> ("delimited string"=w460:string)  [unwired: 9 in]
        n199 = call <userlib>:"1D Array to String__ogtk.vi"("delimiter (Tab)"="\n", "Array of Strings"=w470) -> ("delimited string"=w459:string)  [unwired: 9 in]
        n200 = Format Into String(format string="\n\nConverted File:\n%s\n\nFailed Conversions:\n%s\n\nOriginal Files:\n%s", initial string=w477, error in=w476, w461, w460, w459) -> (resulting string=w474:string, error out=w475:errorcluster)
        n201 = Bundle By Name(cluster=w480, "Log.string"=w474) -> (w479:T3)
        n202 = call <vilib>:"Add State(s) to Queue__JKI_lib_State_Machine.vi"("State(s) in (\"\")"=w482) -> ("States Out"=w481:string)  [unwired: 14 in]
      }
      frame "Log: Write File" {
        # "G:\\My Drive\\ansom\\data\\MNK\\SAMPLE\\"
        # "Experiment Folder--Conversion-Log--DATE.txt"
        # "Experiment"
        # "File"
        # "Your code here.\n(You can make a copy of, or modify, this frame)"
        n203 = Unbundle By Name(w506) -> ("Original"=w501:path[], "Log.Convert End Time"=w495:string, "Log.string"=w492:string)
        "resulting string" <- w492
        n204 = Index Array(array=w501) -> (element=w500:path)  [unwired: 1 in]
        n205 = Strip Path(path=w500) -> (stripped path=w499:path)  [unwired: 1 out]
        n206 = Strip Path(path=w499) -> (stripped path=w503:path, name=w494:string)
        n207 = Format Into String(format string="--Conversion--%s.log" ("name or relative path"), error in=w497, w495) -> (resulting string=w504:string, error out=w496:errorcluster)  [unwired: 1 in]
        n208 = Concatenate Strings(w494, w504) -> (w505:string)
        n209 = Build Path(base path=w503, name or relative path=w505) -> (appended path=w493:path)
        "Log File Path" <- w493
        n210 = Write to Text File(file (use dialog)=w493, text=w492, error in=w496) -> (error out=w502:errorcluster)  [unwired: 1 in, 2 out]
        n211 = call <vilib>:"Add State(s) to Queue__JKI_lib_State_Machine.vi"("State(s) in (\"\")"=w508) -> ("States Out"=w507:string)  [unwired: 14 in]
      }
    }
  }
  "error out" <- w4
  n212 = Unbundle By Name(w2) -> ("Conversion.lvclass"=→"Conversion.lvclass out":refnum<class "Conversion.lvclass">)
